vi "v2.3.vi"() -> ()   [LabVIEW 2018]
uses:
  <vilib>/DAQmx/read.llb/DAQmx Read (Analog 1D DBL NChan 1Samp).vi
  <vilib>/DAQmx/create/channels.llb/DAQmx Create Channel (AI-Temperature-Thermocouple).vi
  <vilib>/DAQmx/configure/timing.llb/DAQmx Timing (Sample Clock).vi
  <vilib>/DAQmx/miscellaneous.llb/DAQmx Fill In Error Info.vi
panel:
  out "Numeric 4":dbl
  out "Numeric 3":dbl
  out "Numeric 2":dbl
  out "Numeric":dbl
  in  "Spectral Amplitude":dbl
  in  "Offset":dbl
  out "Status":T1(ring)
  out "Live Display":dbl[](array[numeric])
  in  "Stop":bool
  in  "OK Button":bool
  in  "DAQ Properties":cluster{"Sample Rate":dbl}={"Sample Rate"=1.0} {"Sample Rate" min=1.0 max=10000.0 step=1.0}
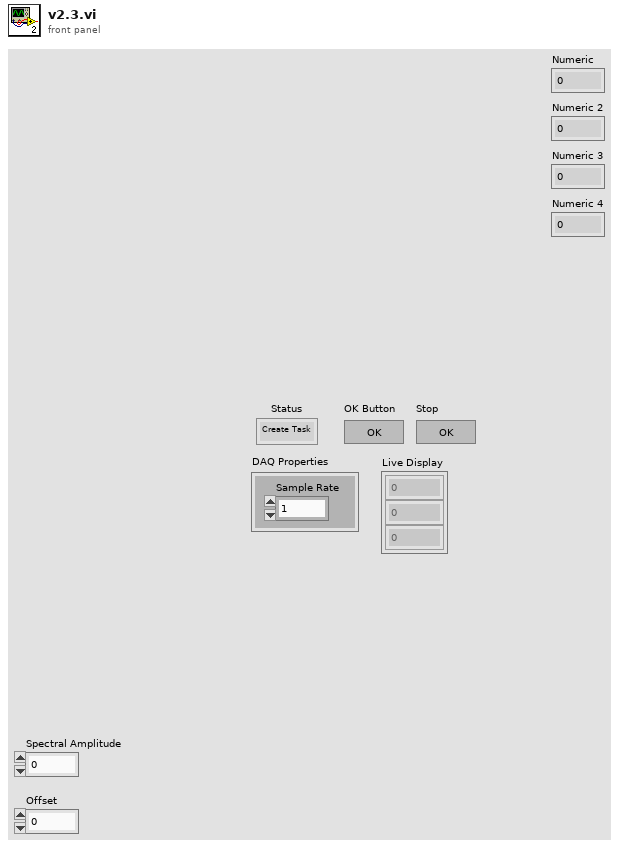
[diagram p1: front panel]
types:
  T1 = enum16{"Create Task", "Change Settings", "Check Settings", "Read Data", "End Task"}
  T2 = enum8{"Enabled", "Disabled", "Disabled and Grayed Out"}
  T3 = cluster{"[0]":dbl, "[1]":dbl, "[2]":dbl, "[3]":dbl}
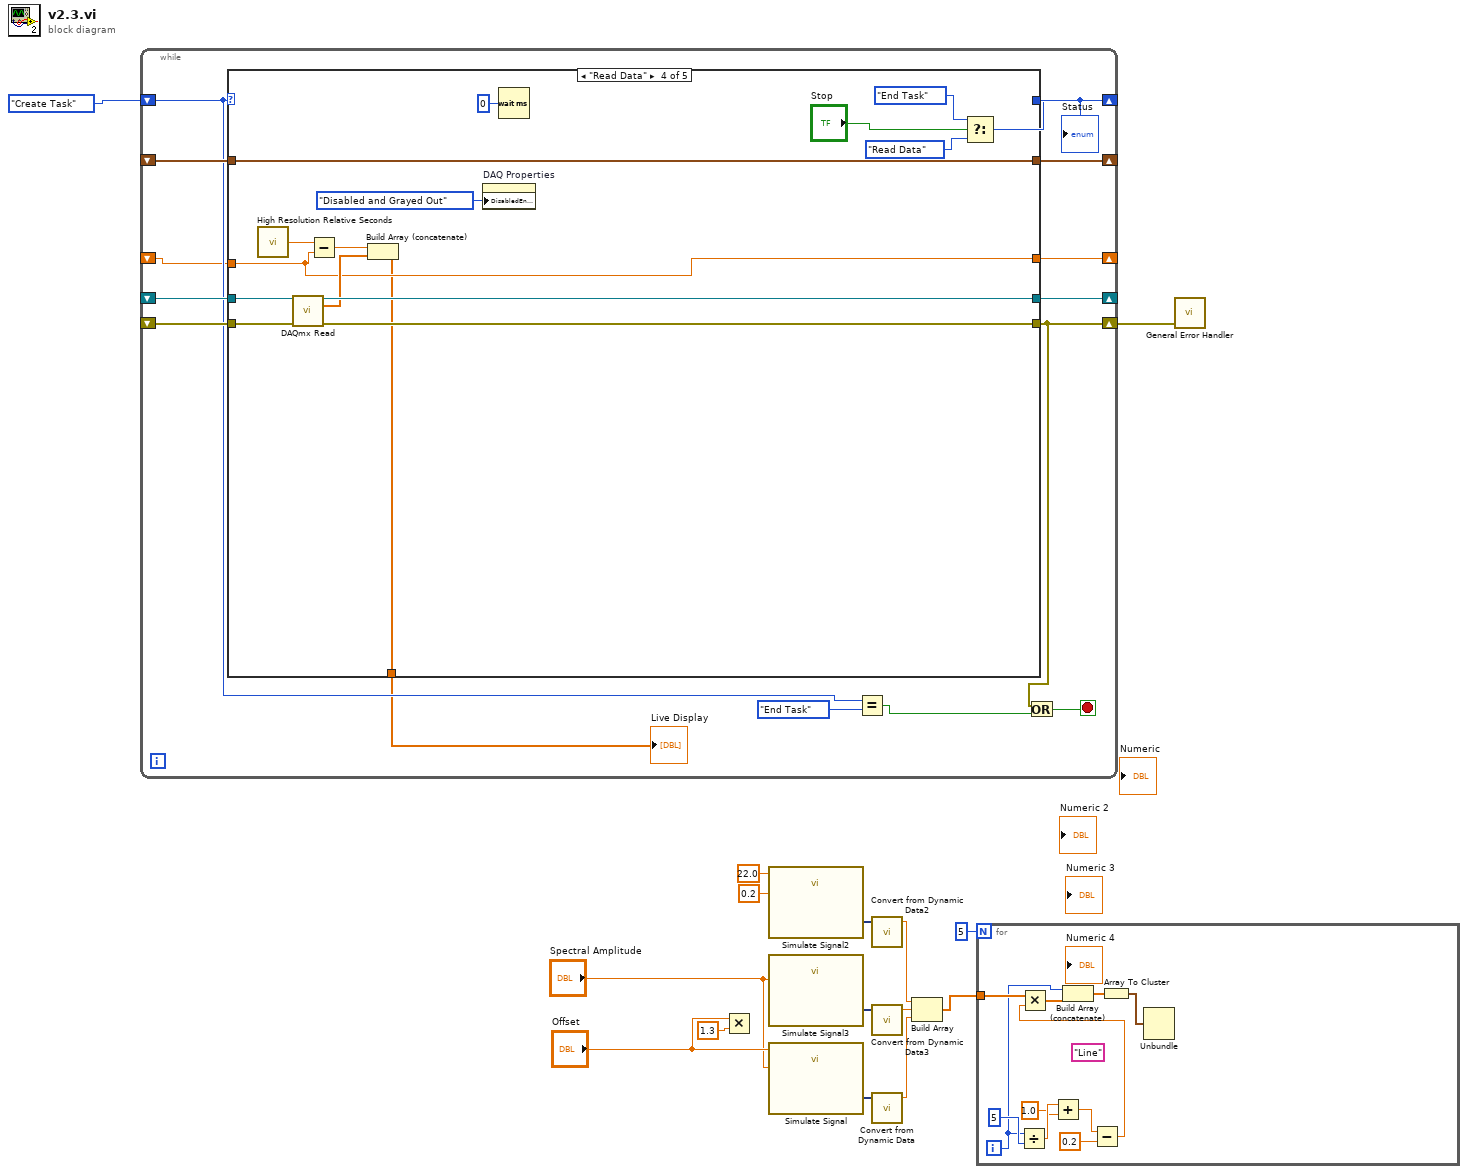
[diagram p0: block diagram]
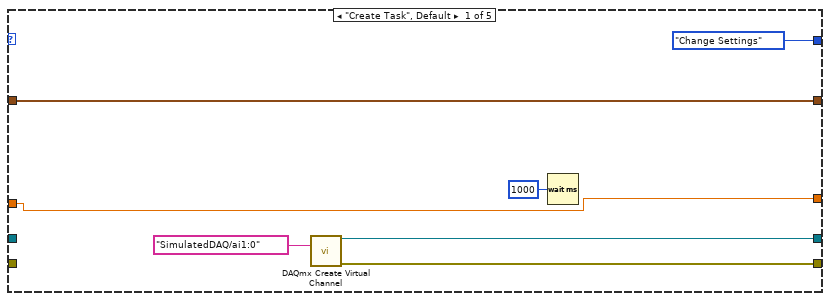
[diagram p2: hidden frame]
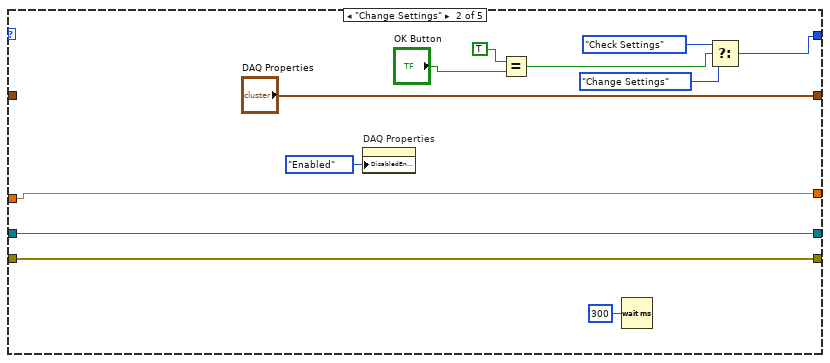
[diagram p3: hidden frame]
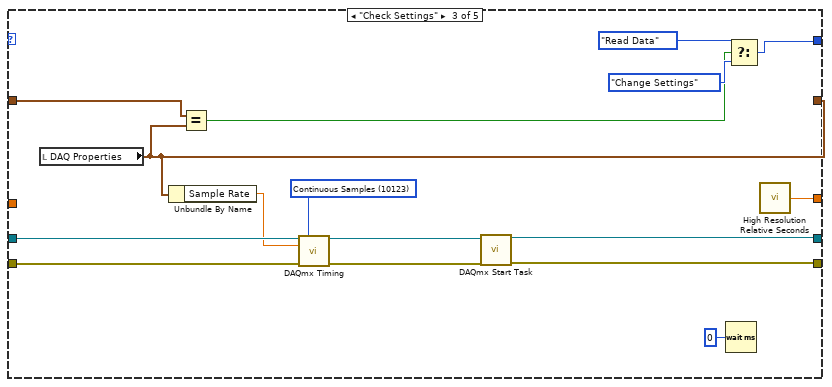
[diagram p4: hidden frame]
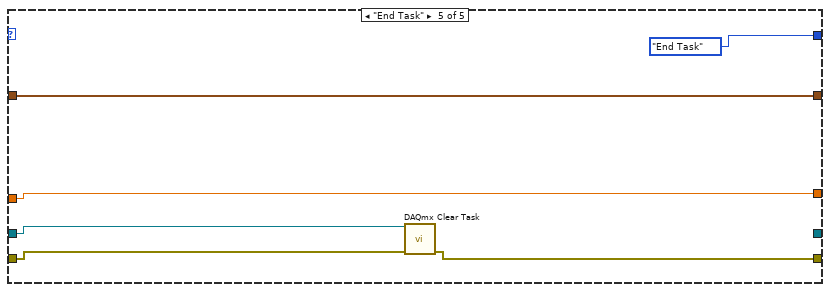
[diagram p5: hidden frame]
diagram:
  n1 = while {
    shift-right: [w24] -> _
    shift-left: T1."Create Task" -> [w19]
    shift-right: [w29] -> _
    shift-left: _ -> [w27]
    shift-right: [w23] -> w14
    shift-left: _ -> [w26]
    shift-right: [w28] -> _
    shift-left: _ -> [w25]
    shift-right: [w18] -> _
    shift-left: _ -> [w17]
    stop <- w22 stop-if-true
    n2 = case shown="\"Read Data\"" w19 {
      tunnel: [w36 w48 w53 w77 _] -> w29
      tunnel: [w35 w47 w52 w76 w86] -> w23
      tunnel: [T1."Change Settings" w41 w60 w74 T1."End Task"] -> w24
      tunnel: [w32 "DAQ Properties" w56 w78 w85] -> w28
      tunnel: w27 -> [_ w48 w59 w80 w83]
      tunnel: w26 -> [_ w47 w58 w79 w82]
      tunnel: w25 -> [w32 _ w64 w78 w85]
      tunnel: [w30 w38 w49 w67 w81] -> w18
      tunnel: w17 -> [w30 w38 _ w67 w81]
      tunnel: [_ _ _ w65 _] -> w16
      frame "Create Task", Default {
        n3 = call-poly <vilib>:"DAQmx Create Virtual Channel.vi"("physical channels"=tag "SimulatedDAQ/ai1:0") -> ("task out"=w36:refnum<k21>, "error out"=w35:errorcluster)  [unwired: 13 in]
        n4 = Wait (ms)(milliseconds to wait=u32 1000) -> ()  [unwired: 1 out]
      }
      frame "Change Settings" {
        n5 = property on="DAQ Properties" class="Clust (strict)"("DisabledEnum"=T2."Enabled" ("Disabled")) -> ()  [unwired: 2 in, 2 out]
        n6 = Equal?(x=TRUE, y="OK Button") -> (x = y?=w43:bool)
        n7 = Wait (ms)(milliseconds to wait=u32 300) -> ()  [unwired: 1 out]
        n8 = Select(t=T1."Check Settings", s=w43, f=T1."Change Settings") -> (s? t:f=w41:T1)
      }
      frame "Check Settings" {
        w50 = 10123 items=["Finite Samples"=10178, "Continuous Samples"=10123, "Hardware Timed Single Point"=12522] ("sample mode")
        n9 = local read "DAQ Properties"() -> (w56:cluster{"Sample Rate":dbl})
        n10 = Unbundle By Name(w56) -> ("Sample Rate"=w57:dbl)
        n11 = Equal?(x=w64, y=w56) -> (x = y?=w51:bool)
        n12 = call-poly <vilib>:"DAQmx Timing.vi"("task/channels in"=w59, "sample mode"=w50, "rate"=w57, "error in"=w58) -> ("task out"=w55:refnum<k21>, "error out"=w54:errorcluster)  [unwired: 10 in]
        n13 = call <vilib>:"DAQmx Start Task.vi"("task/channels in"=w55, "error in"=w54) -> ("task out"=w53:refnum<k21>, "error out"=w52:errorcluster)  [unwired: 12 in]
        n14 = Wait (ms)(milliseconds to wait=u32 0) -> ()  [unwired: 1 out]
        n15 = Select(t=T1."Read Data", s=w51, f=T1."Change Settings") -> (s? t:f=w60:T1)
        n16 = call <vilib>:"High Resolution Relative Seconds.vi"() -> ("relative seconds"=w49:dbl)
      }
      frame "Read Data" {
        n17 = call <vilib>:"High Resolution Relative Seconds.vi"() -> ("relative seconds"=w70:dbl)
        n18 = call-poly <vilib>:"DAQmx Read.vi"("task/channels in"=w80, "error in"=w79) -> ("task out"=w77:refnum<k21>, "data"=w69:dbl[], "error out"=w76:errorcluster)  [unwired: 11 in]
        n19 = Subtract(x=w70, y=w67) -> (x-y=w68:dbl)
        n20 = Build Array (concatenate)(w68, w69) -> (w65:dbl[])
        n21 = property on="DAQ Properties" class="Clust (strict)"("DisabledEnum"=T2."Disabled and Grayed Out" ("Disabled")) -> ()  [unwired: 2 in, 2 out]
        n22 = Wait (ms)(milliseconds to wait=u32 0) -> ()  [unwired: 1 out]
        n23 = Select(t=T1."End Task", s="Stop", f=T1."Read Data") -> (s? t:f=w74:T1)
      }
      frame "End Task" {
        n24 = call <vilib>:"DAQmx Clear Task.vi"("task in"=w83, "error in"=w82) -> ("error out"=w86:errorcluster)  [unwired: 13 in]
      }
    }
    "Live Display" <- w16
    "Status" <- w24
    n25 = Equal?(x=w19, y=T1."End Task") -> (x = y?=w20:bool)
    n26 = Or(x=w23, y=w20) -> (x .or. y?=w22:bool)
  }
  n27 = Multiply(x="Offset", y=1.3) -> ()  [unwired: 1 out]
  n28 = call "Simulate Signal2"("Offset"=22.0, "Spectral amplitude"=0.2) -> ("DC Temperature Signal"=w10:dynamicdata)  [unwired: 12 in, 1 out]
  n29 = call "Simulate Signal3"("Spectral amplitude"="Spectral Amplitude") -> ("DC Pressure Signal"=w11:dynamicdata)  [unwired: 13 in, 1 out]
  n30 = call "Simulate Signal"("Offset"="Offset", "Spectral amplitude"="Spectral Amplitude") -> ("DC Flowrate Signal"=w9:dynamicdata)  [unwired: 12 in, 1 out]
  n31 = call "Convert from Dynamic Data2"("Dynamic Data Type"=w10) -> ("Scalar"=w5:dbl)  [unwired: 3 in]
  n32 = call "Convert from Dynamic Data3"("Dynamic Data Type"=w11) -> ("Scalar"=w4:dbl)  [unwired: 3 in]
  n33 = call "Convert from Dynamic Data"("Dynamic Data Type"=w9) -> ("Scalar"=w3:dbl)  [unwired: 3 in]
  n34 = Build Array(w5, w4, w3) -> (w1:dbl[])
  n35 = for {
    N: 5 -> [_]
    tunnel: w1 -> [w97]
    i -> [w89]
    (unwired) "Line"
    n36 = Divide(x=w89, y=5) -> (x/y=w95:dbl)
    n37 = Add(x=w95, y=1.0) -> (x+y=w93:dbl)
    n38 = Subtract(x=w93, y=0.2) -> (x-y=w91:dbl)
    n39 = Multiply(x=w97, y=w91) -> (x*y=w90:dbl[])
    n40 = Build Array (concatenate)(w89, w90) -> (w88:dbl[])
    n41 = Array To Cluster(array=w88) -> (cluster=w87:T3)
    n42 = Unbundle(w87) -> ()  [unwired: 4 out]
  }
  n43 = call <vilib>:"General Error Handler.vi"("error in (no error)"=w14) -> ()  [unwired: 10 in, 5 out]
